vi "SetRobotProfile.vi"   [LabVIEW 2020]
doc: "Reads the robot profile from the configuration file on the roboRIO."
uses:
  robotprofiles.vi
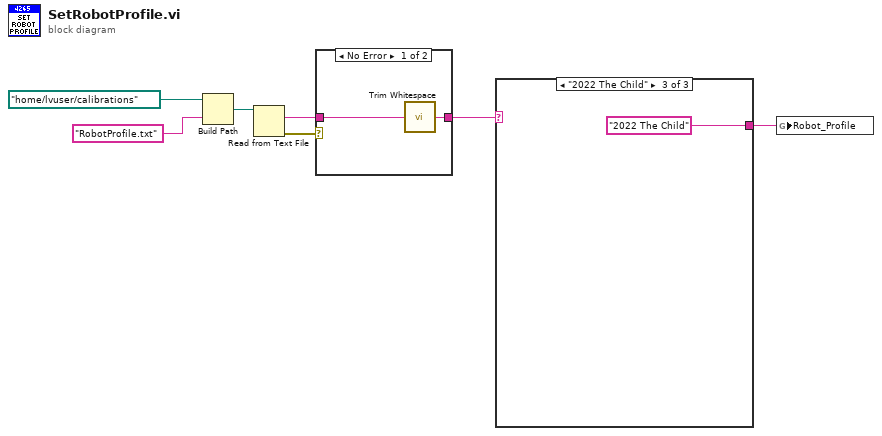
[diagram p0: block diagram]
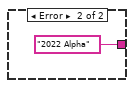
[diagram p2: hidden frame]
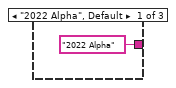
[diagram p3: hidden frame]
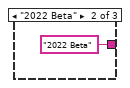
[diagram p4: hidden frame]
diagram:
  n1 = Build Path(base path=path "/home/lvuser/calibrations" ("path"), name or relative path="RobotProfile.txt") -> (appended path=w6:path)
  n2 = Read from Text File(file (use dialog)=w6) -> (text=w4:string, error out=w5:errorcluster)  [unwired: 3 in, 2 out]
  n3 = case shown="No Error" w5 {
    tunnel: w4 -> [w8 _]
    tunnel: [w9 "2022 Alpha"] -> w2
    frame No Error {
      n4 = call <vilib>:"Trim Whitespace.vi"("string"=w8) -> ("trimmed string"=w9:string)  [unwired: 1 in]
    }
    frame Error {
    }
  }
  n5 = case shown="\"2022 The Child\"" w2 {
    tunnel: ["2022 Alpha" "2022 Beta" "2022 The Child"] -> w1
    frame "2022 Alpha", Default {
    }
    frame "2022 Beta" {
    }
    frame "2022 The Child" {
    }
  }
  n6 = global write "robotprofiles.vi" "Robot_Profile"(w1) -> ()
